vi "M_icl_init.vi"() -> (0 "M_icl_init":refnum<queue>)   [LabVIEW 2018]
uses:
  <vilib>/imath/engines/lvmath2/RunTimeEngine/NodeEndStatement/NIMS_NodeEndStatement_Output.vi
  <instcachedir>/0/NIMS_NodeEndStatement_Output_53EC0D466D134D7ABD903AC30B43404B.lvgen/NIMS_NodeEndStatement_Output_53EC0D466D134D7ABD903AC30B43404B_005.vi
  <vilib>/imath/engines/lvmath2/RunTimeEngine/ErrorHandling/NIMS_Finalize Error.vi
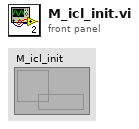
[diagram p1: front panel]
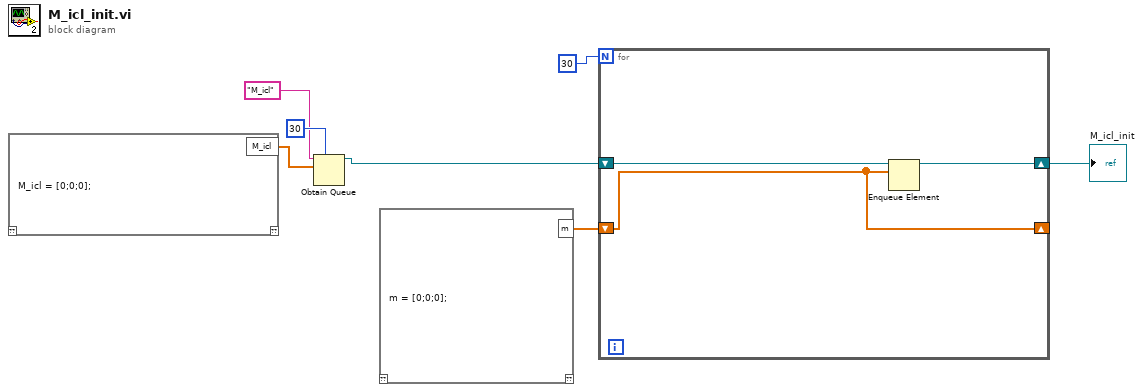
[diagram p0: block diagram]
diagram:
  n1 = mathscript code="M_icl = [0;0;0];"() -> ("M_icl"=w6:dbl[])  [unwired: 1 in, 1 out]
  n2 = Obtain Queue(max queue size (-1, unlimited)=30, name (unnamed)="M_icl", element data type=w6) -> (queue out=w3:refnum<queue>)  [unwired: 2 in, 2 out]
  n3 = mathscript code="m = [0;0;0];"() -> ("m"=w2:dbl[])  [unwired: 1 in, 1 out]
  n4 = for {
    N: 30 -> [_]
    shift-right: [w9] -> w1
    shift-left: w3 -> [w10]
    shift-right: [w8] -> _
    shift-left: w2 -> [w8]
    n5 = Enqueue Element(queue=w10, element=w8) -> (queue out=w9:refnum<queue>)  [unwired: 2 in, 2 out]
  }
  "M_icl_init" <- w1
